vi "StageToStave.vi"() -> ()   [LabVIEW 2016]
panel:
  in  "x change":dbl[](array[numeric])=[-685.0]
  in  "y change":dbl[](array[numeric])=[-55.0]
  in  "z change":dbl[](array[numeric])
  out "Cross- check: Are these the center of pins in the center of the image?":T1[](array[plugin-control])=["image_0", "image_1", "image_2", "image_3", "image_4", "image_5", "image_6", "image_7", "image_8", "image_9", "image_10", "image_11", "image_12", "image_13", "image_14", "image_15", "image_16", "image_17"]
  out "First point (x/y)":dbl[](array[numeric])
  out "Angle of pins":dbl
  out "All average pin coords":dbl[][](array[numeric])
  in  "Captured Coords":path
  out "Check: Plot of average point in each pin":T2(graph)
  in  "Path to save collected images":path=path "C:/Users/Sciolla Lab/Desktop/BNLStaveAssembly-Laura/toolingpins_imagesNew"
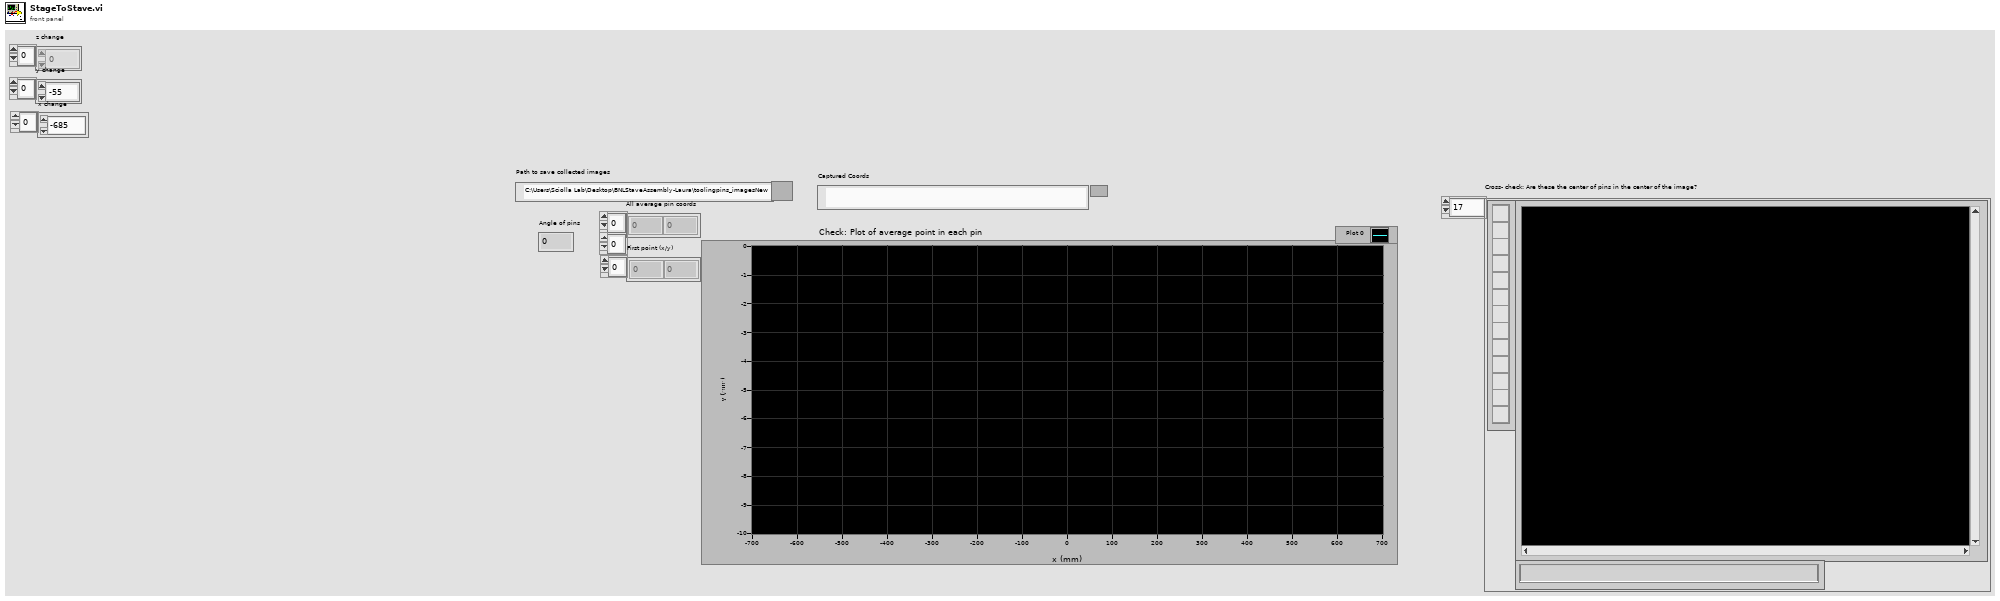
[diagram p1: front panel]
types:
  T1 = typedef "IMAQ Image.ctl" = refnum<image>
  T2 = cluster{"Top averages":dbl[], "Best Linear Fit":dbl[]}[]
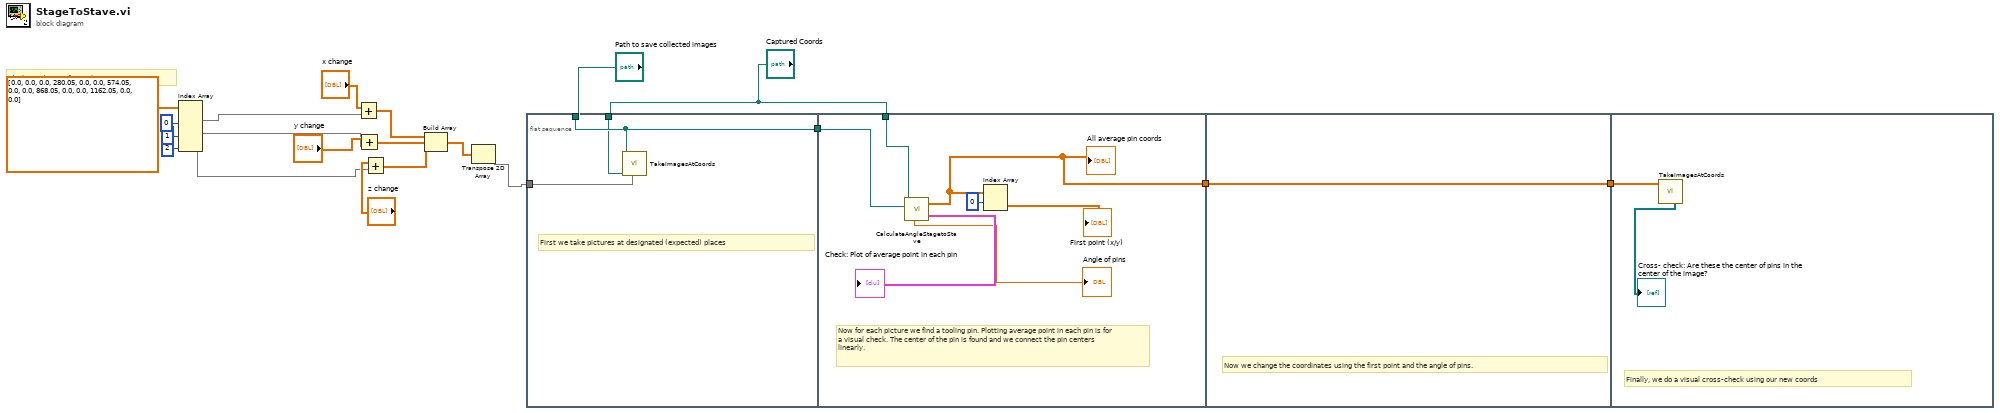
[diagram p0: block diagram]
diagram:
  # "Ideal coordinates for each 5 pins"
  n1 = Index Array(array=dbl[][] [[0.0, 0.0, 0.0], [280.05, 0.0, 0.0], [574.05, 0.0, 0.0], [868.05, 0.0, 0.0], [1162.05, 0.0, 0.0]] ("Set of Coordinates to Process"), index (col) #1=0 ("disabled index (col)"), index (col) #2=1 ("index (col)"), index (col) #3=2 ("index (col)")) -> (element #1=w7:dbl[], element #2=w3:dbl[], element #3=w4:dbl[])  [unwired: 3 in]
  n2 = Add(x="x change", y=w7) -> (x+y=w12:dbl[])
  n3 = Add(x="y change", y=w3) -> (x+y=w11:dbl[])
  n4 = Add(x="z change", y=w4) -> (x+y=w10:dbl[])
  n5 = Build Array(w12, w11, w10) -> (w6:dbl[][])
  n6 = Transpose 2D Array(2D array=w6) -> (transposed array=w5:dbl[][])
  n7 = flat-sequence {
    tunnel: "Path to save collected images" -> [w23]
    tunnel: [w23] -> w19
    tunnel: w5 -> [w22]
    tunnel: "Captured Coords" -> [w21]
    tunnel: w19 -> [w30]
    tunnel: [w25] -> w18
    tunnel: "Captured Coords" -> [w24]
    tunnel: w18 -> [w31]
    tunnel: [w31] -> w17
    tunnel: w17 -> [w32]
    frame #0 {
      # "First we take pictures at designated (expected) places"
      n8 = call "TakeImagesAtCoords.vi"("Set of Coordinates to Process"=w22, "Captured Coords"=w21, "Path to save collected images"=w23) -> ()  [unwired: 8 in, 1 out]
    }
    frame #1 {
      # "Now for each picture we find a tooling pin. Plotting average point in each pin is for a visual check. The center of the pin is found and we connect the pin centers linearly."
      n9 = call "CalculateAngleStagetoStave.vi"("Images Directory"=w30, "Coordinate file for image capture"=w24) -> ("Plot of average point in each pin"=→"Check: Plot of average point in each pin":T2, "First point (x/y)"=w25:dbl[][], "Angle of pins"=→"Angle of pins":dbl)  [unwired: 3 in]
      "All average pin coords" <- w25
      n10 = Index Array(array=w25, index (row)=0) -> (element=→"First point (x/y)":dbl[])  [unwired: 1 in]
    }
    frame #2 {
      # "Now we change the coordinates using the first point and the angle of pins."
    }
    frame #3 {
      # "Finally, we do a visual cross-check using our new coords"
      n11 = call "TakeImagesAtCoords.vi"("Set of Coordinates to Process"=w32) -> ("Image Array"=→"Cross- check: Are these the center of pins in the center of the image?":T1[])  [unwired: 10 in]
    }
  }
